vi "Obtain var refnum.vi"(8 "error in (no error)":errorcluster, 9 "machine name":string, 10 "Humidity var":refnum<k21>, 11 "Temperature var":refnum<k21>) -> (0 "error out":errorcluster, 2 "Humidity Refnum":refnum<k21>, 3 "Temperature Refnum":refnum<k21>)   [LabVIEW 2016]
uses:
  <resource>/objmgr/nvio.rc
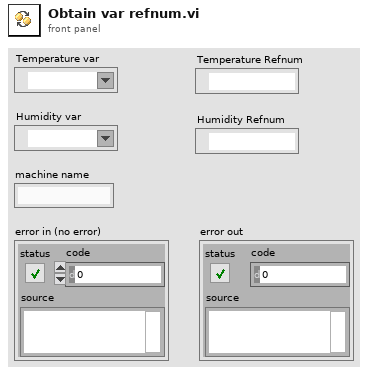
[diagram p1: front panel]
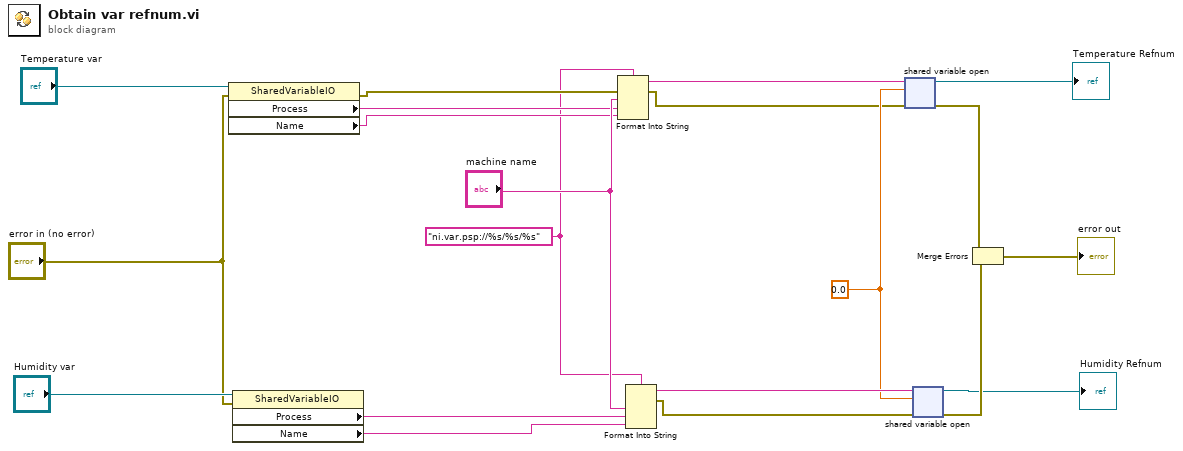
[diagram p0: block diagram]
diagram:
  w1 = "ni.var.psp://%s/%s/%s"
  w6 = 0.0 ("data type")
  n1 = property class="SharedVariableIO"(reference="Temperature var", error in="error in (no error)") -> (error out=w4:errorcluster, "Process"=w8:string, "Name"=w9:string)  [unwired: 1 out]
  n2 = property class="SharedVariableIO"(reference="Humidity var", error in="error in (no error)") -> ("Process"=w10:string, "Name"=w11:string)  [unwired: 2 out]
  n3 = Format Into String(format string=w1, error in=w4, "machine name", w8, w9) -> (resulting string=w13:string, error out=w3:errorcluster)  [unwired: 1 in]
  n4 = Format Into String(format string=w1, "machine name", w10, w11) -> (resulting string=w12:string, error out=w2:errorcluster)  [unwired: 2 in]
  n5 = shared-variable-open(w13, w3, w6) -> (→"Temperature Refnum":refnum<k21>, w19:errorcluster)  [unwired: 1 in]
  n6 = shared-variable-open(w12, w2, w6) -> (→"Humidity Refnum":refnum<k21>, w20:errorcluster)  [unwired: 1 in]
  n7 = Merge Errors(w19, w20) -> (→"error out":errorcluster)
